vi "tester_VI.vi"() -> ()   [LabVIEW 2020]
uses:
  <vilib>/Analysis/Matrix/Datatypes/RealMatrix.ctl
  <vilib>/Analysis/Matrix/Numeric/Conversions/Array To Matrix - RA.vi
  <vilib>/Analysis/Matrix/NI_Matrix.lvlib
panel:
  in  "cell 3 units":dbl
  out "x waveform":dbl(graph)
  out "X":dbl[][](array[numeric])
  in  "X data filepath":path
  in  "cell 2 units":dbl
  in  "cell 1 units":dbl
  out "Array":dbl[][](array[numeric])
  in  "x piecewise tester":T1
  out "y piecewise tester":T1
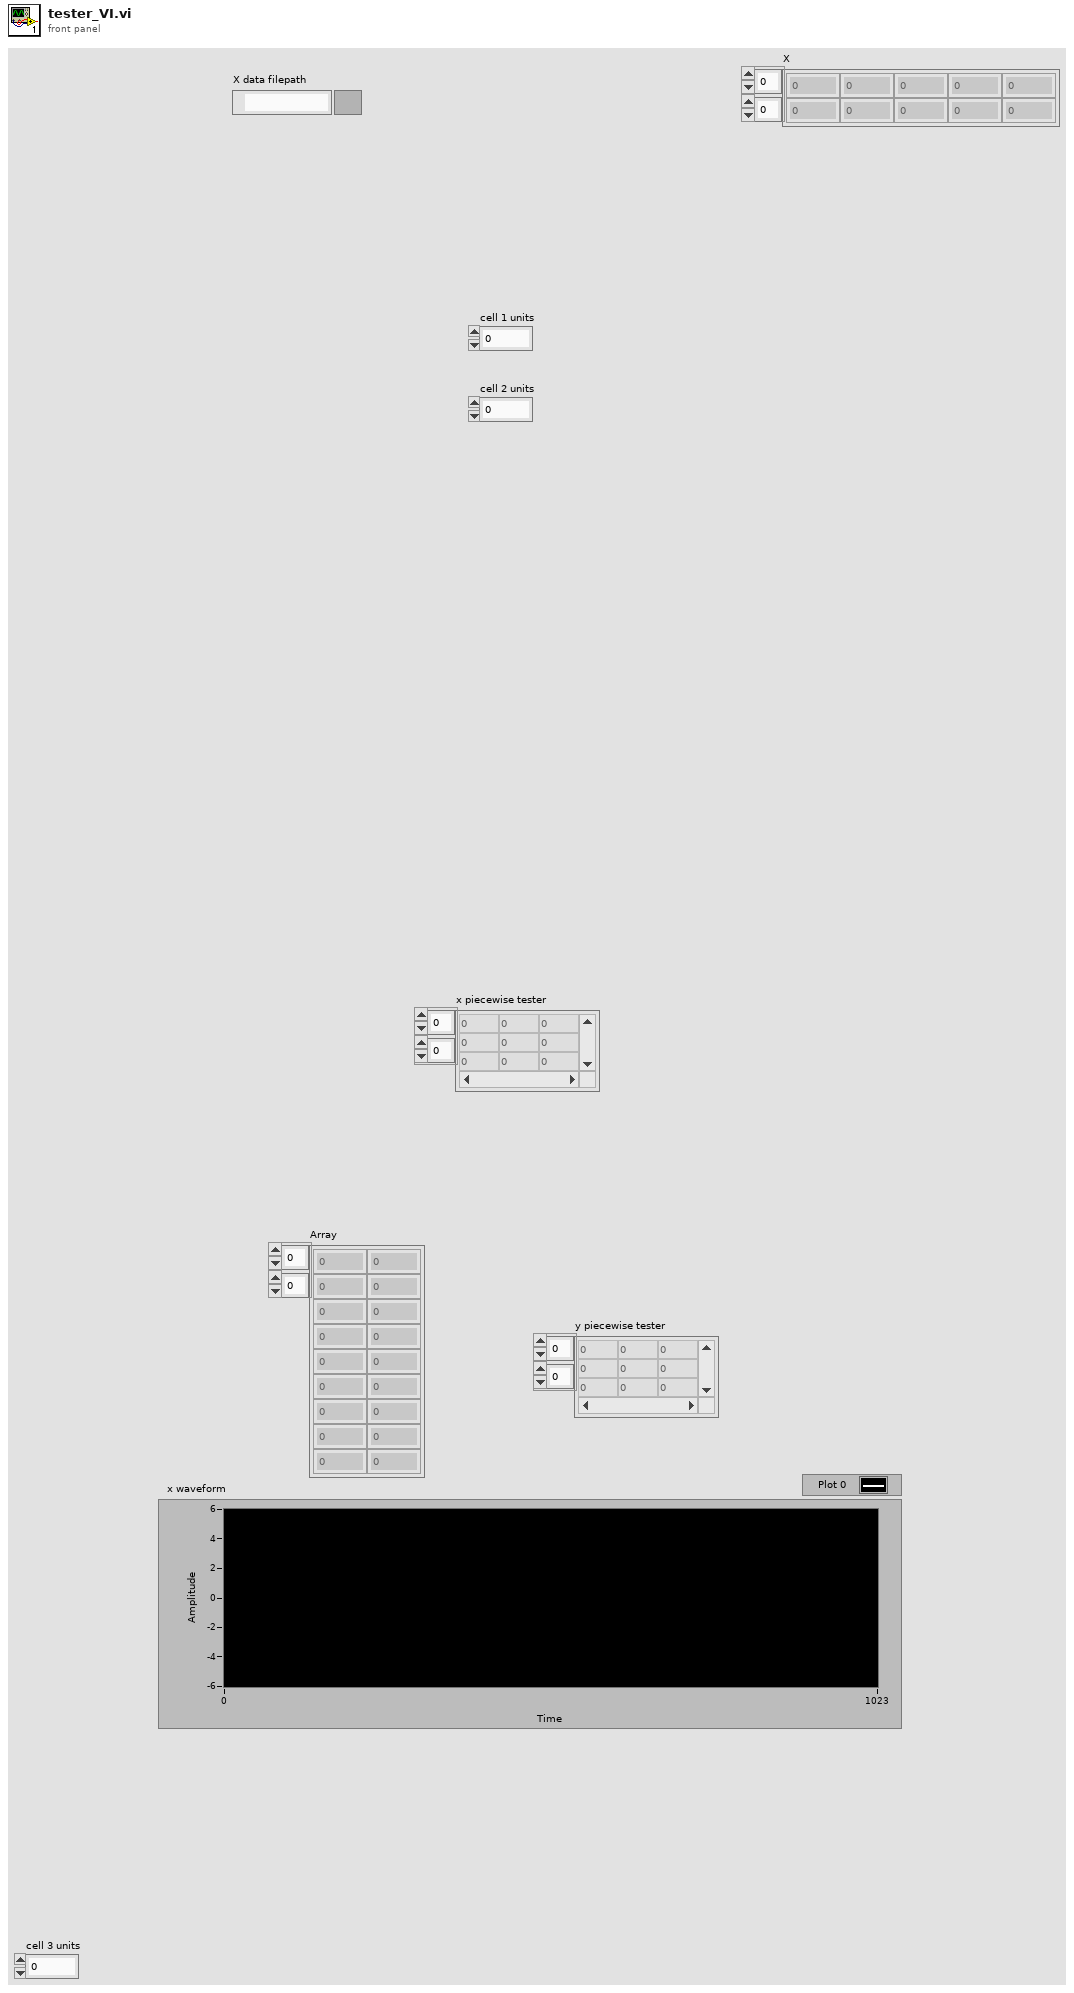
[diagram p1: front panel]
types:
  T1 = typedef "NI_Matrix.lvlib/RealMatrix.ctl" = dbl[][]
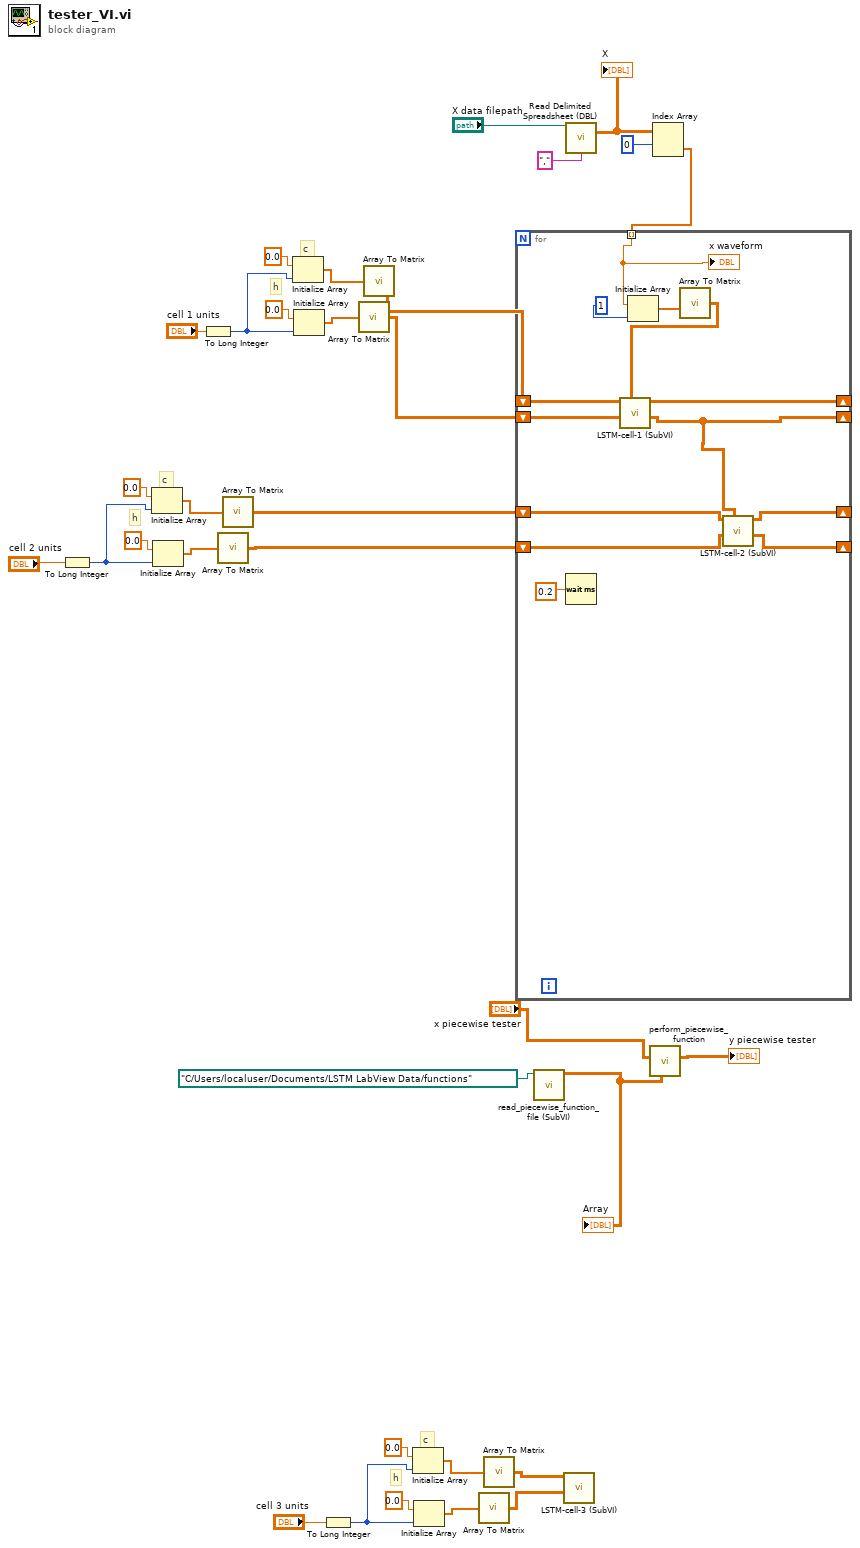
[diagram p0: block diagram]
diagram:
  # "c"
  # "h"
  # "c"
  # "h"
  # "c"
  # "h"
  n1 = To Long Integer(number="cell 2 units") -> (32bit integer=w18:i32)
  n2 = Initialize Array(0.0, w18) -> (w21:dbl[])
  n3 = Initialize Array(0.0, w18) -> (w20:dbl[])
  n4 = To Long Integer(number="cell 1 units") -> (32bit integer=w26:i32)
  n5 = call-poly <vilib>:"Array To Matrix.vi"("Real 1D Array"=w20) -> ("Real Matrix (Column Vector)"=w15:T1)
  n6 = call-poly <vilib>:"Array To Matrix.vi"("Real 1D Array"=w21) -> ("Real Matrix (Column Vector)"=w14:T1)
  n7 = Initialize Array(0.0, w26) -> (w25:dbl[])
  n8 = Initialize Array(0.0, w26) -> (w24:dbl[])
  n9 = To Long Integer(number="cell 3 units") -> (32bit integer=w5:i32)
  n10 = call-poly <vilib>:"Array To Matrix.vi"("Real 1D Array"=w24) -> ("Real Matrix (Column Vector)"=w23:T1)
  n11 = call-poly <vilib>:"Array To Matrix.vi"("Real 1D Array"=w25) -> ("Real Matrix (Column Vector)"=w22:T1)
  n12 = Initialize Array(0.0, w5) -> (w8:dbl[])
  n13 = Initialize Array(0.0, w5) -> (w7:dbl[])
  n14 = call-poly <vilib>:"Array To Matrix.vi"("Real 1D Array"=w7) -> ("Real Matrix (Column Vector)"=w1:T1)
  n15 = call-poly <vilib>:"Array To Matrix.vi"("Real 1D Array"=w8) -> ("Real Matrix (Column Vector)"=w2:T1)
  n16 = call "read_piecewise_function_file (SubVI).vi"("Path"=path "C:/Users/localuser/Documents/LSTM LabView Data/functions") -> ("sigmoid"=w30:dbl[][])  [unwired: 9 in, 1 out]
  "Array" <- w30
  n17 = call "LSTM-cell-3 (SubVI).vi"("h"=w1, "c"=w2) -> ()  [unwired: 8 in, 2 out]
  n18 = call <vilib>:"Read Delimited Spreadsheet (DBL).vi"("file path (dialog if empty)"="X data filepath", "delimiter (\\t)"=",") -> ("all rows"=w11:dbl[][])  [unwired: 8 in, 5 out]
  "X" <- w11
  n19 = call "perform_piecewise_function.vi"("function array"=w30, "x"="x piecewise tester") -> ("y"=→"y piecewise tester":T1)  [unwired: 9 in]
  n20 = Index Array(array=w11, index (row)=0) -> (element=w9:dbl[])  [unwired: 1 in]
  n21 = for {
    tunnel: w9 -> [w35] mode=indexing
    shift-right: [w44] -> _
    shift-left: w22 -> [w45]
    shift-right: [w34] -> _
    shift-left: w23 -> [w46]
    shift-right: [w38] -> _
    shift-left: w14 -> [w39]
    shift-right: [w37] -> _
    shift-left: w15 -> [w40]
    n22 = Wait (ms)(milliseconds to wait=0.2) -> ()  [unwired: 1 out]
    n23 = Initialize Array(w35, 1) -> (w42:dbl[])
    n24 = call-poly <vilib>:"Array To Matrix.vi"("Real 1D Array"=w42) -> ("Real Matrix (Column Vector)"=w41:T1)
    n25 = call "LSTM-cell-1 (SubVI).vi"("x"=w41, "h"=w46, "c"=w45) -> ("h + 1"=w34:T1, "c + 1"=w44:T1)  [unwired: 7 in]
    n26 = call "LSTM-cell-2 (SubVI).vi"("x"=w34, "h"=w40, "c"=w39) -> ("h + 1"=w37:T1, "c + 1"=w38:T1)  [unwired: 7 in]
    "x waveform" <- w35
  }
